vi "Get_Osc_Data.vi"(0 "VISA resource name":refnum<visa-resource-name>="Oscilloscope", 7 "Channel":i32(ring)=4 items=["Channel 1"=1, "Channel 2"=2, "Channel 3"=3, "Channel 4"=4, "Function 1"=5, "Function 2"=6, "Function 3"=7, "Function 4"=8, "Memory 1"=9, "Memory 2"=10, "Memory 3"=11, "Memory 4"=12], 11 "error in":errorcluster, 12 "Amplitude":bool=TRUE, 13 "Width":bool=TRUE, 14 "Delay":bool=TRUE) -> (3 "Amplitude":dbl=0.991, 4 "VISA resource name out":refnum<visa-resource-name>="Oscilloscope", 6 "Width Pos":dbl=9.99999e+37 caption="Width_Pos", 8 "Width Neg":dbl=1.99829e-08 caption="Width_Neg", 10 "Delay":dbl=9.99999e+37 caption="Setup_Time", 15 "error out":errorcluster)   [LabVIEW 2012]
uses:
  C/Program Files/National Instruments/LabVIEW 2012/instr.lib/Agilent 8000 Series/Public/Data/Read Measurement (More).vi
  C/Program Files/National Instruments/LabVIEW 2012/instr.lib/Agilent 8000 Series/Public/Data/Read Measurement (Setup And Hold Time).vi
  C/Program Files/National Instruments/LabVIEW 2012/instr.lib/Agilent 8000 Series/Agilent 8000 Series.lvlib
panel:
  in  "Measurement Function 1b":i32(ring)=17 caption="Measurement Function (0: Rise Time)" items=["Rise Time", "Fall Time", "Frequency", "Period", "Voltage RMS(AC)", "Voltage RMS(DC)", "Voltage RMS (AC,cycle)", "Voltage RMS (DC,cycle)", "Voltage Max", "Voltage Min", "Voltage Middle", "Voltage Vpp", "Voltage High", "Voltage Low", "Voltage Average", "Voltage Average (cycle)", "Width Negative", "Width Positive", "Duty Cycle Positive", "Amplitude", "Overshoot", "Preshoot", "Voltage Base", "Voltage Upper", "Time Max", "Time Min", "Color Grade Crossing", "Color Grade Eye Width", "Color Grade Eye Height", "Color Grade Eye Q-Factory", "Color Grade Eye Duty Cycle Distortion(Percent)", "Color Grade Eye Duty Cycle Distortion(Time)", "Color Grade Eye Jitter(PP)", "Color Grade Eye Width(RMS)", "Cycle-cycle Duty Jitter(Rising)", "Cycle-cycle Duty Jitter(Falling)", "Cycle-cycle Jitter(Rising)", "Cycle-cycle Jitter(Falling)", "Cycle-cycle - Width", "Cycle-cycle + Width", "Date Rate", "Unit Interval", "FFT Delta Frequency", "FFT Delta Magnitude", "FFT Frequency", "FFT Magnitude", "Slew Rate", "Area (Entire Display)", "Area(Single Cycle)", "Duty Cycle (Rising)", "Duty Cycle (Falling)"]
  in  "Measurement Function  2":i32(ring) caption="Measurement Function (0: Setup Time)" items=["Setup Time", "Hold Time"]
  in  "Data Source":u16(ring)=4 caption="Data Source (1: Channel 1)" items=["Channel 1"=1, "Channel 2"=2, "Channel 3"=3, "Channel 4"=4, "Function 1"=5, "Function 2"=6, "Function 3"=7, "Function 4"=8, "Memory 1"=9, "Memory 2"=10, "Memory 3"=11, "Memory 4"=12]
  in  "Clock Source Direction":i32(ring) caption="Clock Source Direction (0: Rising)" items=["Rising", "Falling"]
  in  "Clock Source":u16(ring)=1 caption="Clock Source (2: Channel 2)" items=["Channel 1"=1, "Channel 2"=2, "Channel 3"=3, "Channel 4"=4, "Function 1"=5, "Function 2"=6, "Function 3"=7, "Function 4"=8, "Memory 1"=9, "Memory 2"=10, "Memory 3"=11, "Memory 4"=12]
  in  "Data Source Direction":i32(ring) caption="Data Source Direction (0: Rising)" items=["Rising", "Falling", "Both"]
  in  "Measurement Function 1a":i32(ring)=16 caption="Measurement Function (0: Rise Time)" items=["Rise Time", "Fall Time", "Frequency", "Period", "Voltage RMS(AC)", "Voltage RMS(DC)", "Voltage RMS (AC,cycle)", "Voltage RMS (DC,cycle)", "Voltage Max", "Voltage Min", "Voltage Middle", "Voltage Vpp", "Voltage High", "Voltage Low", "Voltage Average", "Voltage Average (cycle)", "Width Negative", "Width Positive", "Duty Cycle Positive", "Amplitude", "Overshoot", "Preshoot", "Voltage Base", "Voltage Upper", "Time Max", "Time Min", "Color Grade Crossing", "Color Grade Eye Width", "Color Grade Eye Height", "Color Grade Eye Q-Factory", "Color Grade Eye Duty Cycle Distortion(Percent)", "Color Grade Eye Duty Cycle Distortion(Time)", "Color Grade Eye Jitter(PP)", "Color Grade Eye Width(RMS)", "Cycle-cycle Duty Jitter(Rising)", "Cycle-cycle Duty Jitter(Falling)", "Cycle-cycle Jitter(Rising)", "Cycle-cycle Jitter(Falling)", "Cycle-cycle - Width", "Cycle-cycle + Width", "Date Rate", "Unit Interval", "FFT Delta Frequency", "FFT Delta Magnitude", "FFT Frequency", "FFT Magnitude", "Slew Rate", "Area (Entire Display)", "Area(Single Cycle)", "Duty Cycle (Rising)", "Duty Cycle (Falling)"]
  in  "Measurement Function 0":i32(ring)=19 caption="Measurement Function (0: Rise Time)" items=["Rise Time", "Fall Time", "Frequency", "Period", "Voltage RMS(AC)", "Voltage RMS(DC)", "Voltage RMS (AC,cycle)", "Voltage RMS (DC,cycle)", "Voltage Max", "Voltage Min", "Voltage Middle", "Voltage Vpp", "Voltage High", "Voltage Low", "Voltage Average", "Voltage Average (cycle)", "Width Negative", "Width Positive", "Duty Cycle Positive", "Amplitude", "Overshoot", "Preshoot", "Voltage Base", "Voltage Upper", "Time Max", "Time Min", "Color Grade Crossing", "Color Grade Eye Width", "Color Grade Eye Height", "Color Grade Eye Q-Factory", "Color Grade Eye Duty Cycle Distortion(Percent)", "Color Grade Eye Duty Cycle Distortion(Time)", "Color Grade Eye Jitter(PP)", "Color Grade Eye Width(RMS)", "Cycle-cycle Duty Jitter(Rising)", "Cycle-cycle Duty Jitter(Falling)", "Cycle-cycle Jitter(Rising)", "Cycle-cycle Jitter(Falling)", "Cycle-cycle - Width", "Cycle-cycle + Width", "Date Rate", "Unit Interval", "FFT Delta Frequency", "FFT Delta Magnitude", "FFT Frequency", "FFT Magnitude", "Slew Rate", "Area (Entire Display)", "Area(Single Cycle)", "Duty Cycle (Rising)", "Duty Cycle (Falling)"]
  # "Trigger Source"
  # "Setup time Signal"
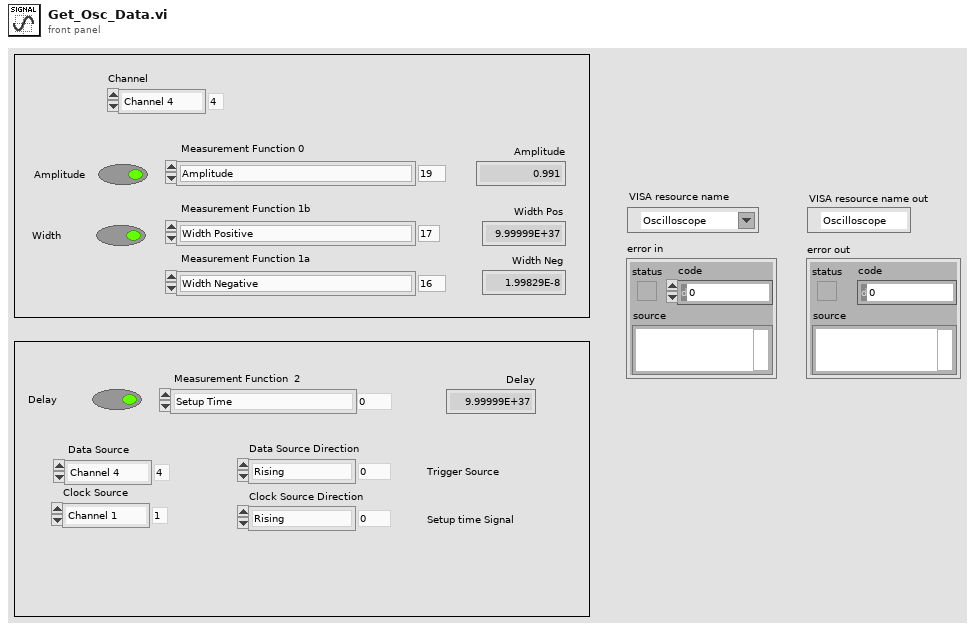
[diagram p1: front panel]
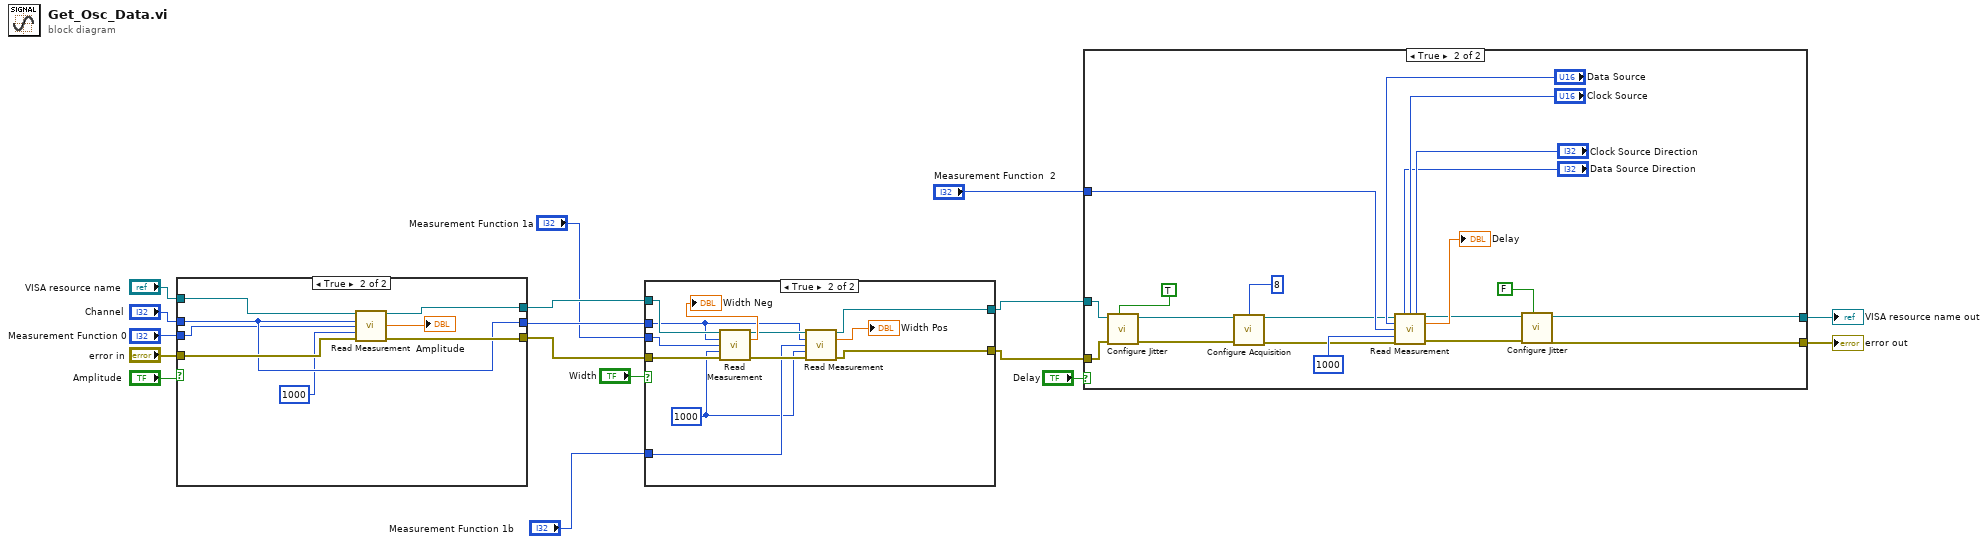
[diagram p0: block diagram]
diagram:
  n1 = case shown="True" "Amplitude" {
    tunnel: "VISA resource name" -> [w20 w25]
    tunnel: "Channel" -> [w18 w23]
    tunnel: "Measurement Function 0" -> [_ w22]
    tunnel: "error in" -> [w19 w24]
    tunnel: [w20 w28] -> w12
    tunnel: [w19 w27] -> w10
    tunnel: [w18 w23] -> w11
    frame False {
    }
    frame True {
      n2 = call-poly "Read Measurement.vi"("VISA resource name"=w25, "Channel (1: Channel 1)"=w23, "Measurement Function (0: Rise Time)"=w22, "Maximum Time (10000ms)"=u32 1000, "error in (no error)"=w24) -> ("VISA resource name out"=w28:refnum<visa-resource-name>, "Measurement"=→"Amplitude":dbl, "error out"=w27:errorcluster)  [unwired: 8 in]
    }
  }
  n3 = case shown="True" "Width" {
    tunnel: w12 -> [w30 w41]
    tunnel: w11 -> [_ w36]
    tunnel: "Measurement Function 1a" -> [_ w40]
    tunnel: w10 -> [w29 w42]
    tunnel: [w30 w33] -> w9
    tunnel: [w29 w32] -> w8
    tunnel: "Measurement Function 1b" -> [_ w35]
    frame False {
    }
    frame True {
      w34 = u32 1000 ("Maximum Time (10000ms)")
      n4 = call-poly "Read Measurement.vi"("VISA resource name"=w41, "Channel (1: Channel 1)"=w36, "Measurement Function (0: Rise Time)"=w40, "Maximum Time (10000ms)"=w34, "error in (no error)"=w42) -> ("VISA resource name out"=w37:refnum<visa-resource-name>, "Measurement"=→"Width Neg":dbl, "error out"=w38:errorcluster)  [unwired: 8 in]
      n5 = call-poly "Read Measurement.vi"("VISA resource name"=w37, "Channel (1: Channel 1)"=w36, "Measurement Function (0: Rise Time)"=w35, "Maximum Time (10000ms)"=w34, "error in (no error)"=w38) -> ("VISA resource name out"=w33:refnum<visa-resource-name>, "Measurement"=→"Width Pos":dbl, "error out"=w32:errorcluster)  [unwired: 8 in]
    }
  }
  n6 = case shown="True" "Delay" {
    tunnel: w9 -> [w43 w56]
    tunnel: w8 -> [w44 w50]
    tunnel: [w44 w51] -> w7
    tunnel: [w43 w52] -> w3
    tunnel: "Measurement Function  2" -> [_ w59]
    frame False {
    }
    frame True {
      n7 = call "Configure Jitter.vi"("Enable Jitter Mode (Enable)"=TRUE, "error in (no error)"=w50, "VISA resource name"=w56) -> ("error out"=w48:errorcluster, "VISA resource name out"=w49:refnum<visa-resource-name>)  [unwired: 7 in]
      n8 = call "Configure Acquisition.vi"("VISA resource name"=w49, "Number Of Averages (8)"=8, "error in (no error)"=w48) -> ("VISA resource name out"=w46:refnum<visa-resource-name>, "error out"=w45:errorcluster)  [unwired: 11 in]
      n9 = call-poly "Read Measurement.vi"("VISA resource name"=w46, "Data Source Direction (0: Rising)"="Data Source Direction", "Clock Source (2: Channel 2)"="Clock Source", "Clock Source Direction (0: Rising)"="Clock Source Direction", "Data Source (1: Channel 1)"="Data Source", "Measurement Function (0: Setup Time)"=w59, "Maximum Time (10000ms)"=u32 1000, "error in (no error)"=w45) -> ("VISA resource name out"=w55:refnum<visa-resource-name>, "Setup or Hold Time (s)"=→"Delay":dbl, "error out"=w54:errorcluster)  [unwired: 5 in]
      n10 = call "Configure Jitter.vi"("Enable Jitter Mode (Enable)"=FALSE, "error in (no error)"=w54, "VISA resource name"=w55) -> ("error out"=w51:errorcluster, "VISA resource name out"=w52:refnum<visa-resource-name>)  [unwired: 7 in]
    }
  }
  "VISA resource name out" <- w3
  "error out" <- w7
